vi "read serial loop.vi"(7 "earth magnetic field":cluster{"x":sgl, "y":sgl, "z":sgl}, 8 "error in (no error)":errorcluster, 9 "disk queues":T1, 10 "display queues":T1, 11 "serial port":refnum<visa-resource-name>) -> (0 "error out":errorcluster, 1 "coil elements read":u32, 2 "re-synch":bool, 3 "VISA resource name out":refnum<visa-resource-name>)   [LabVIEW 2017]
uses:
  typedefs/queue cluster.ctl
  typedefs/reading queue.ctl
  typedefs/reading.ctl
  typedefs/readingType.ctl
  typedefs/reading 1 queue.ctl
  typedefs/reading1.ctl
panel:
  out "synchronized":bool
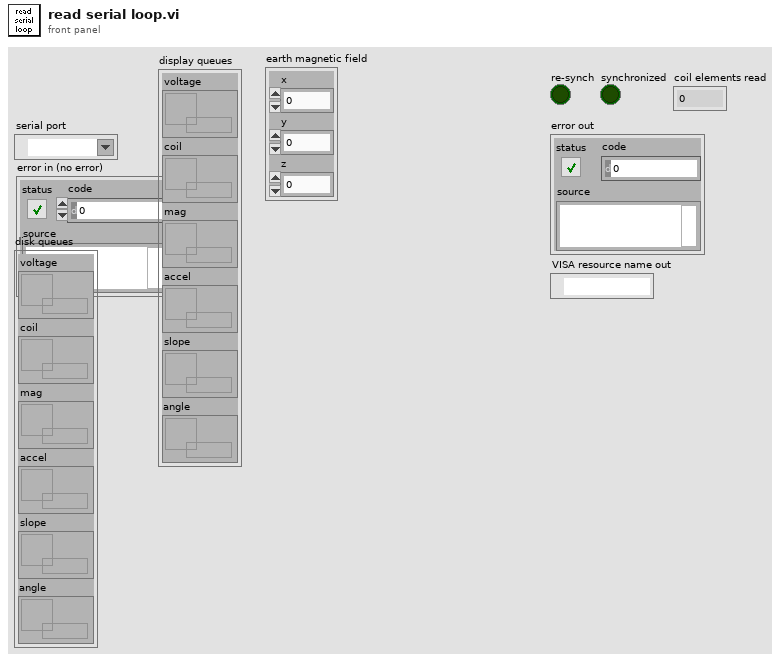
[diagram p1: front panel]
types:
  T1 = typedef "queue cluster.ctl" = cluster{"voltage":T2, "coil":T2, "mag":T2, "accel":T2, "slope":T3, "angle":T2}
  T2 = typedef "reading queue.ctl" = refnum<queue>
  T3 = typedef "reading 1 queue.ctl" = refnum<queue>
  T4 = typedef "reading.ctl" = cluster{"reading type":T5, "time":fxp<+,48,48>, "x":sgl, "y":sgl, "z":sgl, "XSUM":u8}
  T5 = typedef "readingType.ctl" = enum8{"SYNC", "DETVAL", "COILI", "MAGVEC", "ACCVEC"}
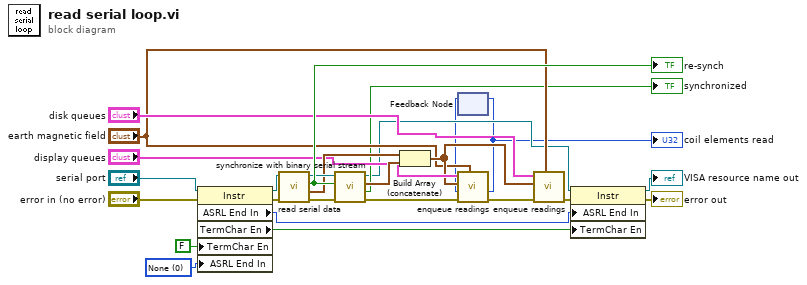
[diagram p0: block diagram]
diagram:
  w10 = u16 0 items=["None", "Last Bit", "TermChar"] ("Serial Settings:End Mode for Reads")
  n1 = property class="Instr"(reference="serial port", error in="error in (no error)", "TermChar En"=FALSE ("Message Based Settings:Termination Character Enable"), "ASRL End In"=w10) -> (reference out=w13:refnum<visa-resource-name>, error out=w9:errorcluster, "ASRL End In"=w4:u16, "TermChar En"=w3:bool)
  n2 = call "read serial data.vi"("error in (no error)"=w9, "serial port"=w13) -> ("error out"=w25:errorcluster, "readings"=w22:T4[], "re-synch"=w24:bool, "serial port out"=w23:refnum<visa-resource-name>)  [unwired: 6 in]
  "re-synch" <- w24
  n3 = call "synchronize with binary serial stream.vi"("error in"=w25, "synch?"=w24, "serial port"=w23) -> ("error out"=w20:errorcluster, "synched?"=→"synchronized":bool, "first reading"=w21:T4, "VISA resource name out"=w8:refnum<visa-resource-name>)  [unwired: 5 in]
  n4 = Build Array (concatenate)(w22, w21) -> (w16:T4[])
  n5 = feedback #1() -> (w1:u32)  [unwired: 1 in]
  n6 = call "enqueue readings.vi"("earth magnetic field"="earth magnetic field", "error in"=w20, "coil elements in"=w1, "readings from serial"=w16, "queues"="display queues") -> ("error out"=w18:errorcluster, "coil elements read"=w2:u32)  [unwired: 5 in]
  "coil elements read" <- w2
  n7 = feedback-in #1(w2) -> ()
  n8 = call "enqueue readings.vi"("earth magnetic field"="earth magnetic field", "error in"=w18, "readings from serial"=w16, "queues"="disk queues") -> ("error out"=w7:errorcluster)  [unwired: 6 in, 1 out]
  n9 = property class="Instr"(reference=w8, error in=w7, "ASRL End In"=w4, "TermChar En"=w3) -> (reference out=→"VISA resource name out":refnum<visa-resource-name>, error out=→"error out":errorcluster)
